vi "dvp Vi Get Trigger Delay.vi"(10 "pTriggerDelay":dbl, 11 "handle":u32) -> (2 "pTriggerDelay out":dbl, 3 "function return":u32(ring))   [LabVIEW 2018, in "LabViewDVPCamera.lvlib"]
doc: "LabviewDvp2Api dvpStatus dvpViGetTriggerDelay(dvpHandle handle, double *pTriggerDelay);"
uses:
  LabViewDVPCamera.lvlib
  LabViewDVPCamera/LabViewDVPCamera.dll
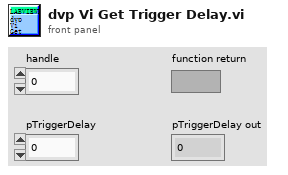
[diagram p1: front panel]
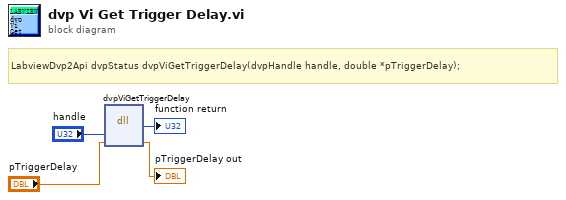
[diagram p0: block diagram]
diagram:
  # "LabviewDvp2Api dvpStatus dvpViGetTriggerDelay(dvpHandle handle, double *pTriggerDelay);"
  n1 = dll-call lib="C:/Program Files (x86)/DVP2 Labview cn 64/Sample/LabViewDVPCamera/LabViewDVPCamera.*" fn="dvpViGetTriggerDelay"("handle"="handle", "pTriggerDelay"="pTriggerDelay") -> (→"function return":u32, "pTriggerDelay"=→"pTriggerDelay out":dbl)  [unwired: 4 in, 2 out]
